vi "Assert Factory Global.vi"(9 "Clear (F)":bool, 10 "Set (F)":bool, 11 "Test Assert Factory in":refnum<class "Test Assert Factory.lvclass">) -> (1 "Is Set?":bool, 2 "Succeeded?":bool, 3 "Test Assert Factory out":refnum<class "Test Assert Factory.lvclass">)   [LabVIEW 2013, in "Caraya.lvlib" / "Assert Factory Manager.lvclass"]
doc: "Stores currently used Assert Factory."
uses:
  Assert Factory Manager.lvclass
  Test Assert Factory/Test Assert Factory.lvclass
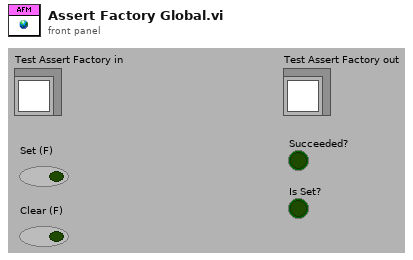
[diagram p1: front panel]
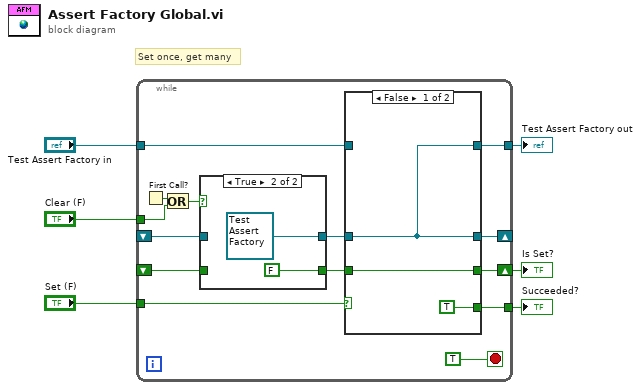
[diagram p0: block diagram]
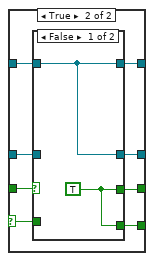
[diagram p3: hidden frame]
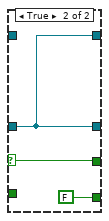
[diagram p4: hidden frame]
diagram:
  # "Set once, get many"
  n1 = while {
    tunnel: "Set (F)" -> [w19]
    tunnel: "Test Assert Factory in" -> [w17]
    shift-right: [w15] -> _
    shift-left: _ -> [w18]
    tunnel: [w14] -> w4
    shift-right: [w12] -> w3
    shift-left: _ -> [w13]
    tunnel: [w10] -> w2
    tunnel: "Clear (F)" -> [w7]
    stop <- TRUE stop-if-true
    n2 = First Call?() -> (First Call?: T/F=w9:bool)
    n3 = Or(x=w9, y=w7) -> (x .or. y?=w8:bool)
    n4 = case shown="True" w8 {
      tunnel: w18 -> [w22 _]
      tunnel: [w22 refnum<class "Test Assert Factory.lvclass"> refnum ("Test Assert Factory")] -> w16
      tunnel: w13 -> [w21 _]
      tunnel: [w21 FALSE] -> w11
      frame False {
      }
      frame True {
      }
    }
    n5 = case shown="False" w19 {
      selector: w19 -> [_ w29]
      tunnel: w17 -> [_ w35]
      tunnel: w16 -> [w27 w32]
      tunnel: [w27 w31] -> w15
      tunnel: [w27 w33] -> w14
      tunnel: [w26 w30] -> w12
      tunnel: w11 -> [w26 w34]
      tunnel: [TRUE w28] -> w10
      frame False {
      }
      frame True {
        n6 = case shown="False" w34 {
          selector: w34 -> [_ w39]
          tunnel: w35 -> [w37 _]
          tunnel: [w37 w40] -> w33
          tunnel: w32 -> [_ w40]
          tunnel: [w37 w40] -> w31
          tunnel: [w36 w39] -> w30
          tunnel: w29 -> [_ _]
          tunnel: [w36 FALSE] -> w28
          frame False {
            w36 = TRUE
          }
          frame True {
          }
        }
      }
    }
  }
  "Test Assert Factory out" <- w4
  "Is Set?" <- w3
  "Succeeded?" <- w2
